vi "txt2bin.vi"() -> ()   [LabVIEW 2014]
uses:
  Type Def/CAN Message.ctl
  <vilib>/Utility/file.llb/Read From Spreadsheet File (string).vi
panel:
  out "Array":u8[](array[numeric])
  out "number of rows":i32
  in  "file path (dialog if empty)":path
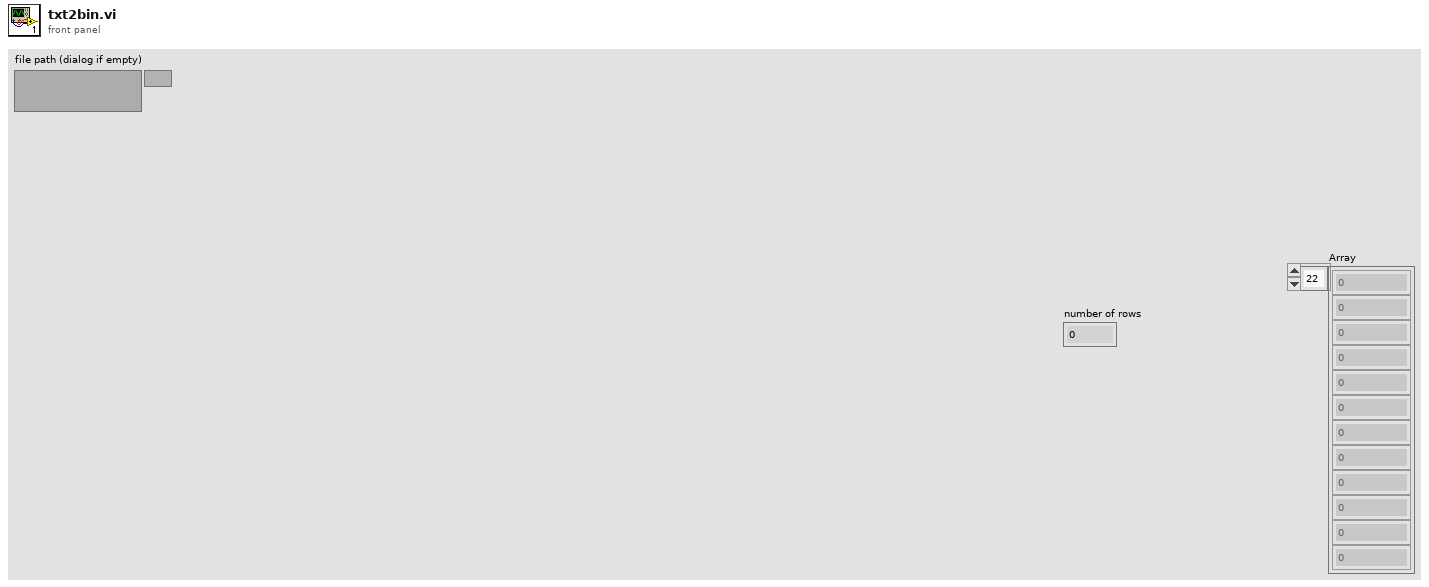
[diagram p1: front panel]
types:
  T1 = typedef "CAN Message.ctl" = cluster{"Msg No.":i32, "Time Dif.":i32, "ID":i32, "DLC":i32, "Message":string}
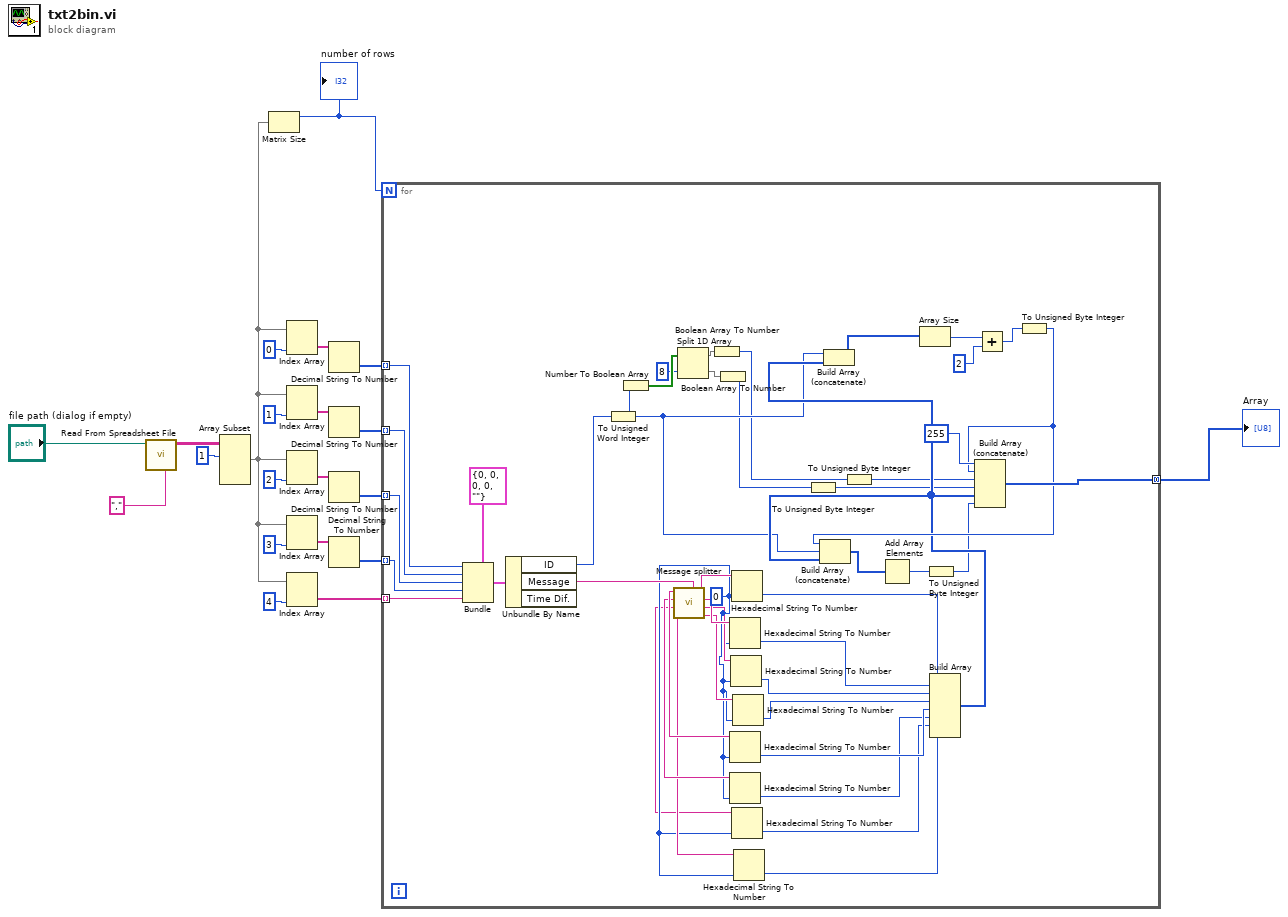
[diagram p0: block diagram]
diagram:
  n1 = call-poly <vilib>:"Read From Spreadsheet File.vi"("delimiter (\\t)"="," ("delimiter (\\t)"), "file path (dialog if empty)"="file path (dialog if empty)") -> ("all rows"=w9:string[][])  [unwired: 5 in, 4 out]
  n2 = Array Subset(array=w9, index (row)=1 ("index")) -> (w19:string[][])  [unwired: 3 in]
  n3 = Matrix Size(0:w19) -> (1:w7:i32)  [unwired: 1 out]
  "number of rows" <- w7
  n4 = Index Array(array=w19, index (col)=0 ("index")) -> (element=w13:string[])  [unwired: 1 in]
  n5 = Index Array(array=w19, index (col)=1 ("index")) -> (element=w12:string[])  [unwired: 1 in]
  n6 = Index Array(array=w19, index (col)=2 ("index")) -> (element=w11:string[])  [unwired: 1 in]
  n7 = Index Array(array=w19, index (col)=3 ("index")) -> (element=w10:string[])  [unwired: 1 in]
  n8 = Index Array(array=w19, index (col)=4 ("index")) -> (element=w2:string[])  [unwired: 1 in]
  n9 = Decimal String To Number(string=w13) -> (number=w6:i32[])  [unwired: 2 in, 1 out]
  n10 = Decimal String To Number(string=w12) -> (number=w5:i32[])  [unwired: 2 in, 1 out]
  n11 = Decimal String To Number(string=w11) -> (number=w4:i32[])  [unwired: 2 in, 1 out]
  n12 = Decimal String To Number(string=w10) -> (number=w3:i32[])  [unwired: 2 in, 1 out]
  n13 = for {
    N: w7 -> [_]
    tunnel: w6 -> [w64] mode=indexing
    tunnel: w5 -> [w65] mode=indexing
    tunnel: w4 -> [w63] mode=indexing
    tunnel: w3 -> [w62] mode=indexing
    tunnel: w2 -> [w61] mode=indexing
    tunnel: [w57] -> w1 mode=concatenating
    w41 = u8 0 ("default (0 U32)")
    n14 = Bundle(cluster=T1 {"Msg No."=0, "Time Dif."=0, "ID"=0, "DLC"=0, "Message"=""}, "Msg No."=w64, "Time Dif."=w65, "ID"=w63, "DLC"=w62, "Message"=w61) -> (w66:T1)
    n15 = Unbundle By Name(w66) -> ("ID"=w60:i32, "Message"=w50:string)  [unwired: 1 out]
    n16 = To Unsigned Word Integer(number=w60) -> (unsigned 16bit integer=w30:u16)
    n17 = Number To Boolean Array(number=w30) -> (Boolean array=w29:bool[])
    n18 = call "Message splitter.vi"("Message in"=w50) -> ("Byte 4"=w45:string, "Byte 3"=w46:string, "Byte 2"=w47:string, "Byte 1"=w49:string, "Byte 8"=w42:string, "Byte 7"=w32:string, "Byte 6"=w43:string, "Byte 5"=w44:string)  [unwired: 3 in]
    n19 = Split 1D Array(array=w29, index=8) -> (first subarray=w27:bool[], second subarray=w26:bool[])
    n20 = Boolean Array To Number(Boolean array=w27) -> (number=w25:u32)
    n21 = Boolean Array To Number(Boolean array=w26) -> (number=w24:u32)
    n22 = Hexadecimal String To Number(string=w47, default (0uL)=w41) -> (number=w39:u8)  [unwired: 1 in, 1 out]
    n23 = Hexadecimal String To Number(string=w44, default (0uL)=w41) -> (number=w36:u8)  [unwired: 1 in, 1 out]
    n24 = Hexadecimal String To Number(string=w43, default (0uL)=w41) -> (number=w35:u8)  [unwired: 1 in, 1 out]
    n25 = Hexadecimal String To Number(string=w46, default (0uL)=w41) -> (number=w38:u8)  [unwired: 1 in, 1 out]
    n26 = Hexadecimal String To Number(string=w49, default (0uL)=w41) -> (number=w40:u8)  [unwired: 1 in, 1 out]
    n27 = Hexadecimal String To Number(string=w32, default (0uL)=w41) -> (number=w34:u8)  [unwired: 1 in, 1 out]
    n28 = Hexadecimal String To Number(string=w45, default (0uL)=w41) -> (number=w37:u8)  [unwired: 1 in, 1 out]
    n29 = Hexadecimal String To Number(string=w42, default (0uL)=w41) -> (number=w33:u8)  [unwired: 1 in, 1 out]
    n30 = To Unsigned Byte Integer(number=w24) -> (unsigned 8bit integer=w22:u8)
    n31 = To Unsigned Byte Integer(number=w25) -> (unsigned 8bit integer=w23:u8)
    n32 = Build Array(w40, w39, w38, w37, w36, w35, w34, w33) -> (w48:u8[])
    n33 = Build Array (concatenate)(w30, w48) -> (w59:u16[])
    n34 = Array Size(array=w59) -> (size(s)=w54:i32)
    n35 = Add(x=w54, y=2) -> (x+y=w55:i32)
    n36 = To Unsigned Byte Integer(number=w55) -> (unsigned 8bit integer=w53:u8)
    n37 = Build Array (concatenate)(w53, w30, w48) -> (w52:u16[])
    n38 = Add Array Elements(numeric array=w52) -> (sum=w51:u16)
    n39 = To Unsigned Byte Integer(number=w51) -> (unsigned 8bit integer=w31:u8)
    n40 = Build Array (concatenate)(u8 255, w53, w23, w22, w48, w31) -> (w57:u8[])
  }
  "Array" <- w1
